vi "Init.vi"(8 "error in (no error)":errorcluster, 11 "UI Actor in":refnum<class "UI Actor.lvclass">) -> (0 "error out":errorcluster, 3 "UI Actor out":refnum<class "UI Actor.lvclass">)   [LabVIEW 2019, in "UI Actor.lvlib" / "UI Actor.lvclass"]
uses:
  UI Actor.lvclass
  C:/Program Files/National Instruments/LabVIEW 2019/vi.lib/ActorFramework/Actor/Actor.lvclass
  UI Actor.lvclass/UI Actor.ctl
  MXN Actor/MXN Actor.lvclass
  MXN Actor/MXN Actor.lvclass/MXN Actor.ctl
  USD Actor/USD Actor.lvclass
  USD Actor/USD Actor.lvclass/USD Actor.ctl
  Bakery Actor/Bakery Actor.lvclass
  Bakery Actor/Bakery Actor.lvclass/Bakery Actor.ctl
  Coffee Actor/Coffee Actor.lvclass
  Coffee Actor/Coffee Actor.lvclass/Coffee Actor.ctl
  Read Coins.vi
  Read Sub Panel Coin.vi
  Read Products.vi
  Read Sub Panel Prod.vi
  <vilib>/ActorFramework/Actor/Actor.lvclass
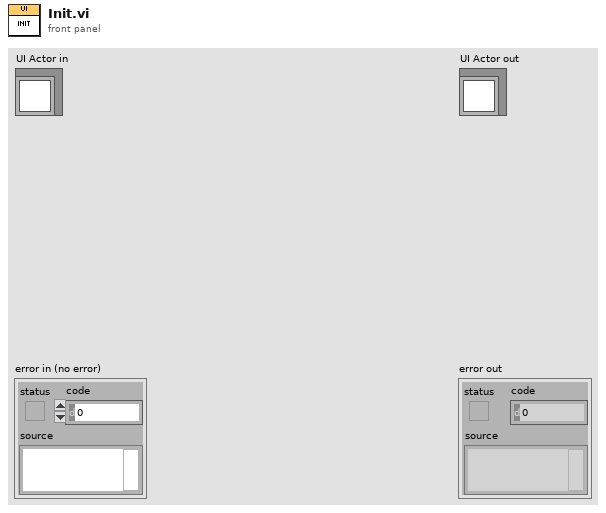
[diagram p1: front panel]
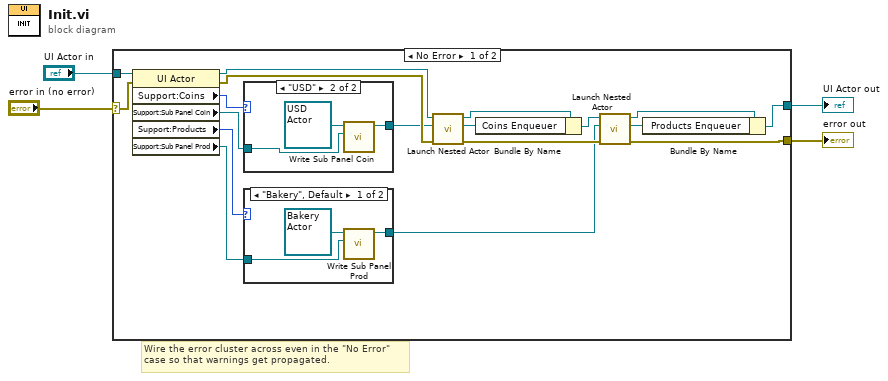
[diagram p0: block diagram]
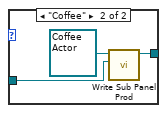
[diagram p2: hidden frame]
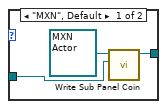
[diagram p3: hidden frame]
diagram:
  # "Wire the error cluster across even in the \"No Error\"\ncase so that warnings get propagated."
  n1 = case shown="No Error" "error in (no error)" {
    selector: "error in (no error)" -> [w21 w36]
    tunnel: [w19 w36] -> w3
    tunnel: [w17 w35] -> w1
    tunnel: "UI Actor in" -> [w22 w35]
    frame No Error {
      n2 = property class="UI Actor"(reference=w22, error in=w21) -> (reference out=w10:refnum<class "UI Actor.lvclass">, error out=w12:errorcluster, "Support:Coins"=w20:enum16{"MXN", "USD"}, "Support:Sub Panel Coin"=w15:refnum<vi>, "Support:Products"=w14:enum16{"Bakery", "Coffee"}, "Support:Sub Panel Prod"=w13:refnum<vi>)
      n3 = case shown="\"USD\"" w20 {
        tunnel: [w30 w33] -> w6
        tunnel: w15 -> [w29 w32]
        frame "MXN", Default {
          n4 = call "Write Sub Panel Coin.vi"("Sub Panel Coin"=w29, "MXN Actor in"=refnum<class "MXN Actor.lvclass"> refnum ("MXN Actor.lvlib:MXN Actor.lvclass")) -> ("MXN Actor out"=w30:refnum<class "MXN Actor.lvclass">)  [unwired: 8 in, 1 out]
        }
        frame "USD" {
          n5 = call "Write Sub Panel Coin.vi"("Sub Panel Coin"=w32, "USD Actor in"=refnum<class "USD Actor.lvclass"> refnum ("USD Actor.lvlib:USD Actor.lvclass")) -> ("USD Actor out"=w33:refnum<class "USD Actor.lvclass">)  [unwired: 8 in, 1 out]
        }
      }
      n6 = case shown="\"Bakery\", Default" w14 {
        tunnel: [w24 w27] -> w5
        tunnel: w13 -> [w23 w26]
        frame "Bakery", Default {
          n7 = call "Write Sub Panel Prod.vi"("Sub Panel Prod"=w23, "Bakery Actor in"=refnum<class "Bakery Actor.lvclass"> refnum ("Bakery Actor.lvlib:Bakery Actor.lvclass")) -> ("Bakery Actor out"=w24:refnum<class "Bakery Actor.lvclass">)  [unwired: 8 in, 1 out]
        }
        frame "Coffee" {
          n8 = call "Write Sub Panel Prod.vi"("Sub Panel Prod"=w26, "Coffee Actor in"=refnum<class "Coffee Actor.lvclass"> refnum ("Coffee Actor.lvlib:Coffee Actor.lvclass")) -> ("Coffee Actor out"=w27:refnum<class "Coffee Actor.lvclass">)  [unwired: 8 in, 1 out]
        }
      }
      n9 = call <vilib>:"Launch Nested Actor.vi"("error in (no error)"=w12, "Nested Actor"=w6, "Caller Actor in"=w10) -> ("error out"=w11:errorcluster, "Nested Actor's Enqueuer"=w9:refnum<class "Message Enqueuer.lvclass">, "Caller Actor out"=w8:refnum<class "UI Actor.lvclass">)  [unwired: 6 in]
      n10 = Bundle By Name(cluster=w8, "Coins Enqueuer"=w9) -> (w7:refnum<class "UI Actor.lvclass">)
      n11 = call <vilib>:"Launch Nested Actor.vi"("error in (no error)"=w11, "Nested Actor"=w5, "Caller Actor in"=w7) -> ("error out"=w19:errorcluster, "Nested Actor's Enqueuer"=w16:refnum<class "Message Enqueuer.lvclass">, "Caller Actor out"=w18:refnum<class "UI Actor.lvclass">)  [unwired: 6 in]
      n12 = Bundle By Name(cluster=w18, "Products Enqueuer"=w16) -> (w17:refnum<class "UI Actor.lvclass">)
    }
    frame Error {
    }
  }
  "error out" <- w3
  "UI Actor out" <- w1
